vi "TaskForJoyStick_ControlMessage.vi"(8 "error in (no error)":errorcluster caption="错误输入（无错误）", 10 "con_手动控制簇":cluster{"Buttons":T1, "All Axis":T11}, 11 "Actor in":refnum<class "ControlPanel.lvclass">) -> (0 "error out":errorcluster caption="错误输出", 3 "Actor out":refnum<class "ControlPanel.lvclass">)   [LabVIEW 2014, in "ControlPanel.lvlib" / "ControlPanel.lvclass"]
uses:
  ControlPanel.lvclass
  <vilib>/MakerHub/Xbox-One-Controller/Private/Type Defs/Indicators/All Buttons Visual.ctl
  <vilib>/MakerHub/Xbox-One-Controller/Private/Type Defs/Indicators/A.ctl
  <vilib>/MakerHub/Xbox-One-Controller/Private/Type Defs/Indicators/B.ctl
  <vilib>/MakerHub/Xbox-One-Controller/Private/Type Defs/Indicators/X.ctl
  <vilib>/MakerHub/Xbox-One-Controller/Private/Type Defs/Indicators/Y.ctl
  <vilib>/MakerHub/Xbox-One-Controller/Private/Type Defs/Indicators/Left Bumper.ctl
  <vilib>/MakerHub/Xbox-One-Controller/Private/Type Defs/Indicators/Right Bumper.ctl
  <vilib>/MakerHub/Xbox-One-Controller/Private/Type Defs/Indicators/View.ctl
  <vilib>/MakerHub/Xbox-One-Controller/Private/Type Defs/Indicators/Menu.ctl
  <vilib>/MakerHub/Xbox-One-Controller/Private/Type Defs/Indicators/Thumbstick.ctl
  <vilib>/MakerHub/Xbox-One-Controller/Private/Type Defs/Indicators/All Axis Data.ctl
  <vilib>/MakerHub/Xbox-One-Controller/Private/Type Defs/Indicators/DPad Enum.ctl
  ControlPanel.lvclass/ControlPanel.ctl
  <vilib>/MakerHub/Xbox-One-Controller/LMH-Xbox-One-Controller.lvlib
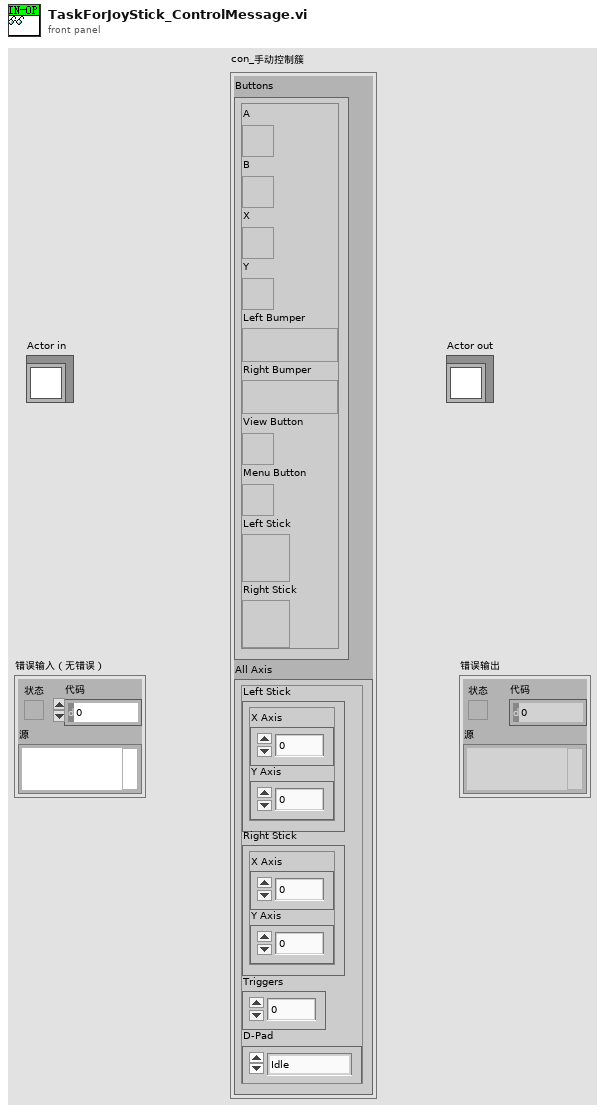
[diagram p1: front panel]
types:
  T1 = typedef "LMH-Xbox-One-Controller.lvlib/All Buttons Visual.ctl" = cluster{"A":T2, "B":T3, "X":T4, "Y":T5, "Left Bumper":T6, "Right Bumper":T7, "View Button":T8, "Menu Button":T9, "Left Stick":T10, "Right Stick":T10}
  T2 = typedef "LMH-Xbox-One-Controller.lvlib/A.ctl" = bool
  T3 = typedef "LMH-Xbox-One-Controller.lvlib/B.ctl" = bool
  T4 = typedef "LMH-Xbox-One-Controller.lvlib/X.ctl" = bool
  T5 = typedef "LMH-Xbox-One-Controller.lvlib/Y.ctl" = bool
  T6 = typedef "LMH-Xbox-One-Controller.lvlib/Left Bumper.ctl" = bool
  T7 = typedef "LMH-Xbox-One-Controller.lvlib/Right Bumper.ctl" = bool
  T8 = typedef "LMH-Xbox-One-Controller.lvlib/View.ctl" = bool
  T9 = typedef "LMH-Xbox-One-Controller.lvlib/Menu.ctl" = bool
  T10 = typedef "LMH-Xbox-One-Controller.lvlib/Thumbstick.ctl" = bool
  T11 = typedef "LMH-Xbox-One-Controller.lvlib/All Axis Data.ctl" = cluster{"Left Stick":cluster{"X Axis":i32, "Y Axis":i32}, "Right Stick":cluster{"X Axis":i32, "Y Axis":i32}, "Triggers":i32, "D-Pad":T12}
  T12 = typedef "LMH-Xbox-One-Controller.lvlib/DPad Enum.ctl" = enum16{"Idle", "Up", "Up / Right", "Right", "Down / Right", "Down", "Down / Left", "Left", "Up / Left"}
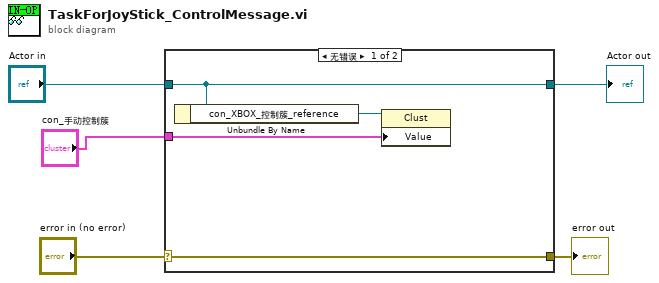
[diagram p0: block diagram]
diagram:
  n1 = case shown="无错误" "error in (no error)" {
    selector: "error in (no error)" -> [w9 w10]
    tunnel: [w9 w10] -> w4
    tunnel: [w8 w11] -> w1
    tunnel: "Actor in" -> [w8 w11]
    tunnel: "con_手动控制簇" -> [w6 _]
    frame No Error {
      n2 = Unbundle By Name(w8) -> ("con_XBOX_控制簇_reference"=w7:refnum<vi>)
      n3 = property class="Clust"(reference=w7, "Value"=w6) -> ()  [unwired: 1 in, 2 out]
    }
    frame Error {
    }
  }
  "error out" <- w4
  "Actor out" <- w1
